vi "Read TLV RAW STR Payload.vi"(8 "error in (no error)":errorcluster, 9 "Length":u8, 11 "object in":refnum<class "CAN IO.lvclass">) -> (0 "error out":errorcluster, 2 "TLV Payload":string, 3 "object out":refnum<class "CAN IO.lvclass">)   [LabVIEW 2013, in "CAN IO.lvclass"]
uses:
  CAN IO.lvclass
  CAN IO.lvclass/CAN IO.ctl
panel:
  out "offset (in bytes)":i64
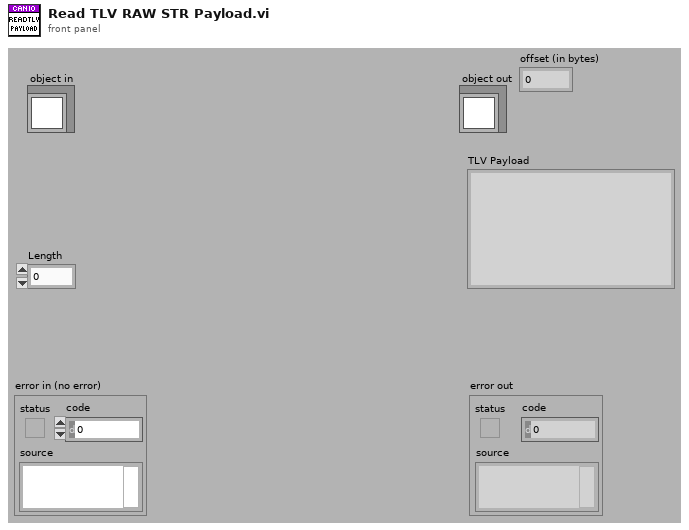
[diagram p1: front panel]
types:
  T1 = enum16{"big-endian, network order", "native, host order", "little-endian"}
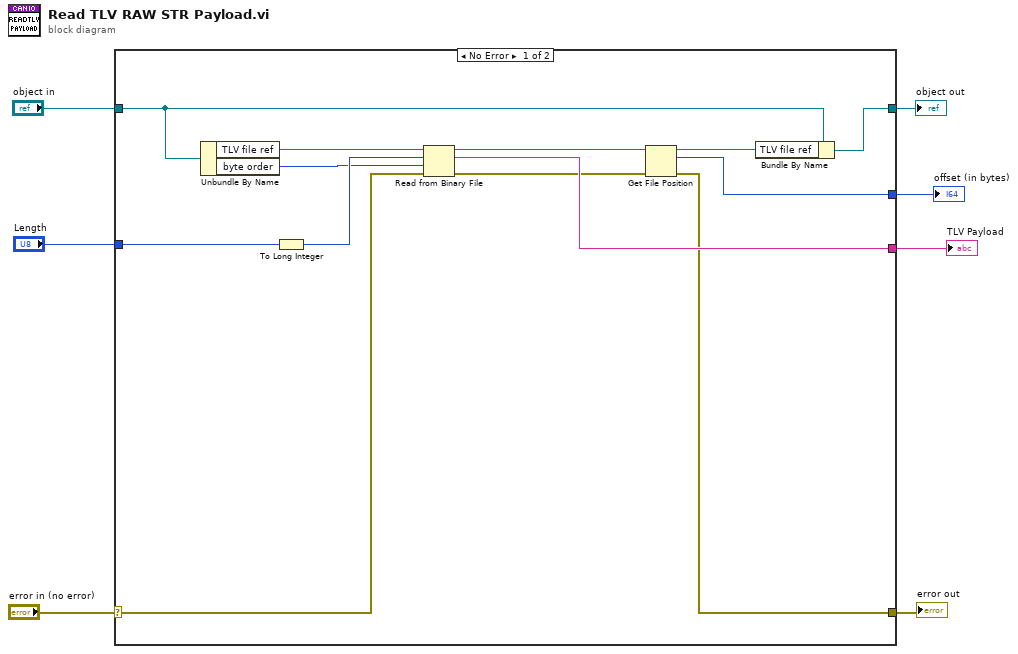
[diagram p0: block diagram]
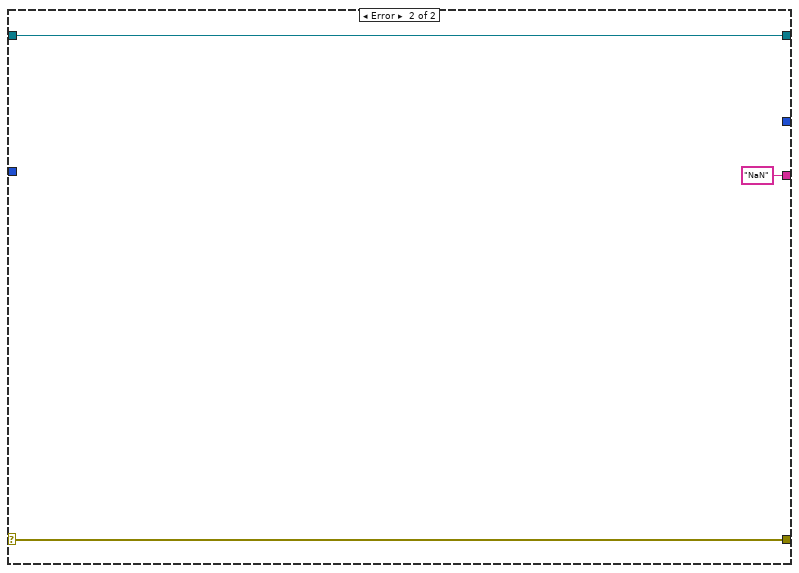
[diagram p2: hidden frame]
diagram:
  n1 = case shown="No Error" "error in (no error)" {
    selector: "error in (no error)" -> [w16 w23]
    tunnel: [w8 w23] -> w6
    tunnel: [w13 w22] -> w4
    tunnel: "object in" -> [w14 w22]
    tunnel: "Length" -> [w19 _]
    tunnel: [w15 "NaN"] -> w2
    tunnel: [w10 _] -> w1
    frame No Error {
      n2 = Unbundle By Name(w14) -> ("TLV file ref"=w20:refnum<file>, "byte order"=w17:T1)
      n3 = To Long Integer(number=w19) -> (32bit integer=w18:i32)
      n4 = Read from Binary File(8:w16, 9:w17, 10:w18, 11:w20) -> (0:w9:errorcluster, 2:w15:string, 3:w12:refnum<file>)  [unwired: 2 in, 1 out]
      n5 = Get File Position(4:w9, 7:w12) -> (0:w8:errorcluster, 2:w10:i64, 3:w11:refnum<file>)
      n6 = Bundle By Name(cluster=w14, "TLV file ref"=w11) -> (w13:refnum<class "CAN IO.lvclass">)
    }
    frame Error {
    }
  }
  "error out" <- w6
  "object out" <- w4
  "TLV Payload" <- w2
  "offset (in bytes)" <- w1
